vi "Process.vi"(8 "error in":errorcluster, 11 "Inst UI.Xeryon-Rotator":refnum<class "Inst UI.Xeryon-Rotator.lvclass">) -> (0 "error out":errorcluster, 3 "Inst UI.Xeryon-Rotator out":refnum<class "Inst UI.Xeryon-Rotator.lvclass">)   [LabVIEW 2019, in "Inst UI.Xeryon-Rotator.lvclass"]
doc: "---------------------------------------------------------------\nJKI State Machine Objects™\nhttp://jki.net/state-machine-objects/\nCopyright (C) 2005-2015, JKI <info@jki.net>\nALL RIGHTS RESERVEDJKI State Machine Objects (SMO) 1.0.0.5\nJKI - JKI\nCopyright (c) 2016, JKI"
uses:
  Inst UI.Xeryon-Rotator.lvclass
  C:/Program Files (x86)/National Instruments/LabVIEW 2019/vi.lib/JKI/JKI SMO/SMO/SMO.lvclass
  C:/Program Files (x86)/National Instruments/LabVIEW 2019/user.lib/LevyLab/Instrument Framework/Instrument UI/Instrument UI.lvclass
  C:/Program Files (x86)/National Instruments/LabVIEW 2019/vi.lib/JKI/JKI SMO/SMO.UI/SMO.UI.lvclass
  <userlib>/LevyLab/Instrument Framework/Instrument Types/Cryostat/Typedefs/setAngle--cluster.ctl
  Inst.Xeryon-Rotator/Typedefs/Inst.Xeryon-Rotator.ScanState--Enum.ctl
  Inst.Xeryon-Rotator/Typedefs/Inst.Xeryon-Rotator.getAll--Cluster.ctl
  Inst.Xeryon-Rotator/Inst.Xeryon-Rotator.lvclass
  C:/Program Files (x86)/National Instruments/LabVIEW 2019/user.lib/LevyLab/Instrument Framework/Instrument/Instrument.lvclass
  Inst UI.Xeryon-Rotator.UI--Cluster.ctl
  <userlib>/LevyLab/Configuration/Configuration.lvclass
  <userlib>/LevyLab/RemoteControl/RemoteControl/Typedefs/Message--Cluster.ctl
  <userlib>/LevyLab/Instrument Framework/Instrument UI/Instrument UI.lvclass/Instrument UI.ctl
  Inst.Xeryon-Rotator/Inst.Xeryon-Rotator.lvclass/Inst.Xeryon-Rotator.ctl
  <vilib>/JKI/JKI SMO/SMO/SMO.lvclass/SMO.ctl
  <userlib>/LevyLab/Configuration/Configuration.lvclass/Configuration.ctl
  <userlib>/LevyLab/Instrument Framework/Instrument/Typedefs/Client Type--Enum.ctl
  <userlib>/LevyLab/Instrument Framework/Instrument/Instrument.lvclass/Instrument.ctl
  e9f0865c-66ad-4c19-bb34-0e698946f1b4.vi
  fbc1e19e-d7b2-448f-8f6c-080fe6692cf7.vi
  2b403158-dc38-43e7-94d2-04ca50d476d7.vi
  2b5fa6da-c280-4914-92c0-3208c3c43a45.vi
  20157899-4549-4947-8324-d0895f4678d5.vi
  cd4b701c-744b-455d-abd0-f4a1a0a0dcf1.vi
  <vilib>/JKI/JKI SMO/SMO/Private/ReftoDVR--SMO.vi
  cd4b701c-744b-455d-abd0-f4a1a0a0dcf1.vi/5058294c-336d-4b2b-804e-8f9495cbe216.vi
  cd4b701c-744b-455d-abd0-f4a1a0a0dcf1.vi/49ec677a-2f26-4dd4-a9e7-83f22994531d.vi
  <vilib>/JDP Science/JSONtext/Variant to JSON Text.vi
  <vilib>/Utility/Data Type/Get Type Information.vi
  <vilib>/JDP Science/JSONtext/JSON text to Variant.vi
  <userlib>/LevyLab/Instrument Framework/Instrument/API/Instrument.sendMessageToProcess (string).vi
  <vilib>/JDP Science/JSONtext/LVClass Serializer/JSONtext LVClass Serializer.lvclass
  <userlib>/LevyLab/Instrument Framework/Instrument/Instrument.lvclass
  <userlib>/LevyLab/Instrument Framework/Instrument UI/Instrument UI.lvclass
  <userlib>/LevyLab/RemoteControl/RemoteControl/RemoteControl.lvclass
  C:/Program Files (x86)/National Instruments/LabVIEW 2019/user.lib/LevyLab/Instrument Framework/Instrument Types/Cryostat/Instrument.Cryostat.lvclass
  <userlib>/LevyLab/Instrument Framework/Instrument Types/Cryostat/Instrument.Cryostat.lvclass
  <vilib>/JKI/JKI SMO/SMO/SMO.lvclass
  <vilib>/JKI/JKI SMO/SMO.UI/SMO.UI.lvclass
panel:
  in  "Reset":bool
  out "STAT":string
  in  "Rotate Right":bool
  in  "Rotate Left":bool
  in  "Stop":bool
  out "Color Box":u32(colorbox)
  in  "Rate (°/min)":dbl=1000.0
  out "Waveform Chart":T1(graph)
  out "Position Reached":bool
  out "Right Limit":bool
  out "Left Limit":bool
  out "Index Found":bool
  out "Encoder Position (encoder units)":dbl format="%#_8f"
  out "Desired Position (encoder units)":dbl format="%#_8f"
  out "Encoder Position (°)":dbl
  out "Desired Position (°)":dbl
  out "Numeric":u32
  in  "Go To Position":bool
  in  "Desired Position (°)":dbl
  # "SMO UI Template"
  # "For instructions on how to use the JKI State Machine Objects, examples and video tutorials, visit:\nhttp://jki.net/state-machine-objects/\n\nJKI State Machine Objects™\nhttp://jki.net/state-machine-objects/\nCopyright (C) 2005-2015, JKI <info@jki.net>\nALL RIGHTS RESERVED"
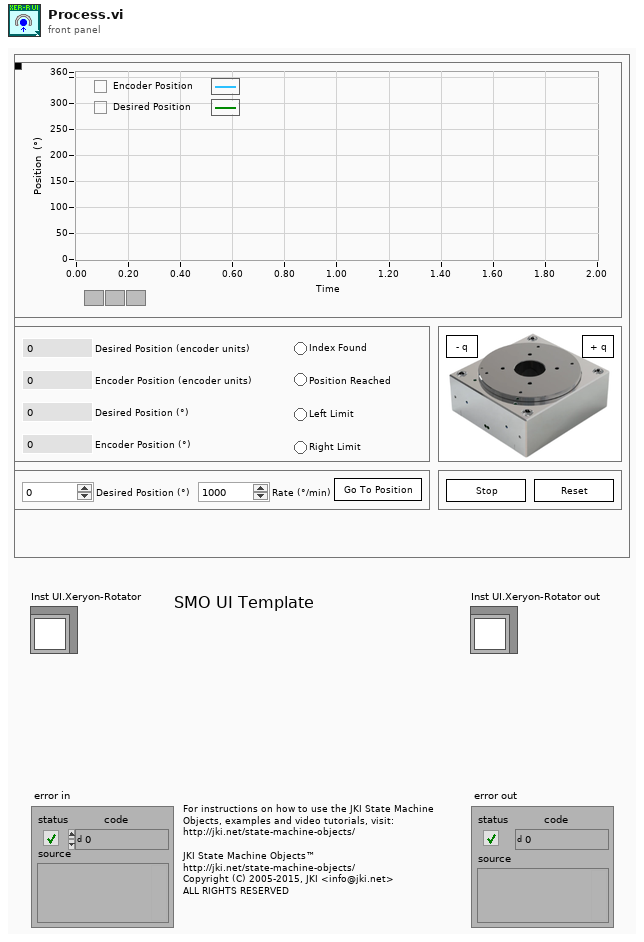
[diagram p1: front panel]
types:
  T1 = cluster{"DPOS In Current Units":dbl, "EPOS In Current Units":dbl}
  T2 = typedef "Instrument.Cryostat.lvclass/setAngle--cluster.ctl" = cluster{"angle":dbl, "rate":dbl, "channel":i32}
  T3 = typedef "Inst.Xeryon-Rotator.lvclass/Inst.Xeryon-Rotator.ScanState--Enum.ctl" = enum16{"Scan Left", "Stop", "Scan Right", "Reset"}
  T4 = enum32{"invalid app kind", "Development System", "Run Time System", "Student Edition", "Embedded LabVIEW", "Evaluation", "Custom"}
  T5 = typedef "Inst.Xeryon-Rotator.lvclass/Inst.Xeryon-Rotator.getAll--Cluster.ctl" = cluster{"Encoder position [selected units]":dbl, "Desired Position [selected units]":dbl, "Status":string, "SRNO":dbl, "SOFT":dbl, "STAT":dbl, "FREQ":dbl, "OFRQ":dbl, "CURR":dbl, "SYNC":dbl, "Encoder Position [enc. units]":dbl, "Desired Position [enc. units]":dbl, "TIME":dbl, "Index Found":bool, "Left Limit":bool, "Right Limit":bool, "Position Reached":bool}
  T6 = enum32{"Invalid", "Standard", "Closed", "Hidden", "Minimized", "Maximized"}
  T7 = typedef "Instrument.lvlib/Instrument.lvclass/Client Type--Enum.ctl" = enum16{"Remote", "Local"}
  T8 = typedef "Inst UI.Xeryon-Rotator.lvclass/Inst UI.Xeryon-Rotator.UI--Cluster.ctl" = cluster{"Desired Position":dbl, "Desired Rate":dbl}
  T9 = typedef "RemoteControl.lvlib/RemoteControl.lvclass/Message--Cluster.ctl" = cluster{"Command":string, "Data":variant, "ID":string, "error":errorcluster}
  T10 = cluster{"Core":cluster{"Current VI Reference":refnum<vi>, "Close Panel on Exit?":bool, "Last Error":cluster{"error":errorcluster, "previous state":string, "remaining states":string}, "Shutdown?":bool}, "Instrument UI":refnum<class "Inst UI.Xeryon-Rotator.lvclass">, "Instrument":refnum<class "Inst.Xeryon-Rotator.lvclass">, "Configuration":refnum<class "Configuration.lvclass">, "getAll":T5, "UI Cluster":T8, "Message":T9}
  T11 = cluster{"Current VI Reference":refnum<vi>, "Close Panel on Exit?":bool, "Last Error":cluster{"error":errorcluster, "previous state":string, "remaining states":string}, "Shutdown?":bool}
  T12 = cluster{"Encoder position [selected units]":dbl, "Desired Position [selected units]":dbl}
  T13 = typedef "SMO.lvclass/Protected Events.ctl" = cluster{"StopProcesses":refnum<user-event>, "AbortProcesses":refnum<user-event>, "Config Changed":refnum<user-event>, "Dependency":refnum<user-event>}
  T14 = typedef "Instrument.lvlib/Instrument.lvclass/PublicEvents--Cluster.ctl" = cluster{"MessageFromProcess":refnum<user-event>}
  T15 = typedef "Inst.Xeryon-Rotator.lvclass/PublicEvents--Cluster.ctl" = cluster{"MessageFromProcess":refnum<user-event>}
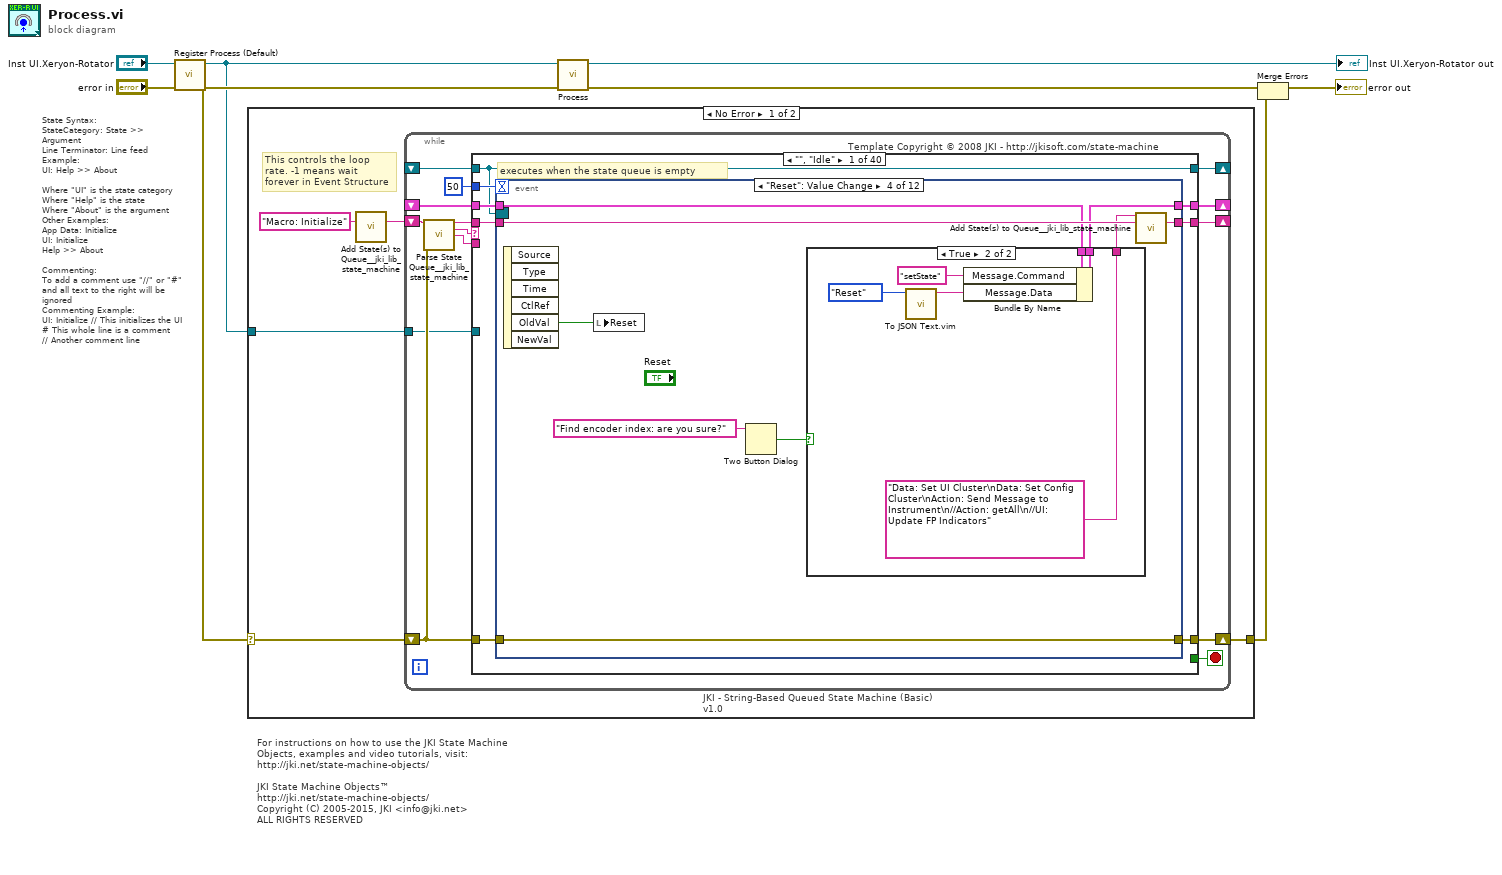
[diagram p0: block diagram]
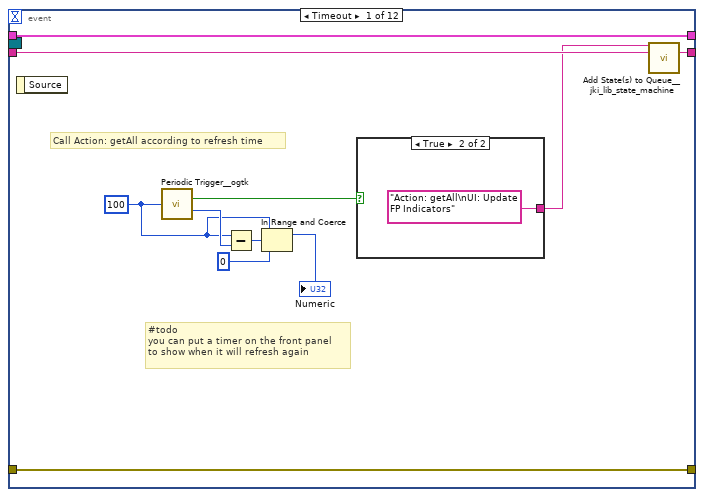
[diagram p2: hidden frame]
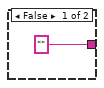
[diagram p3: hidden frame]
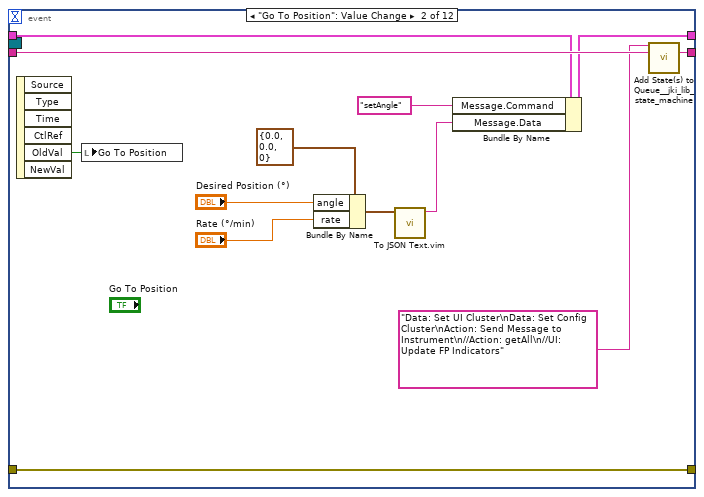
[diagram p4: hidden frame]
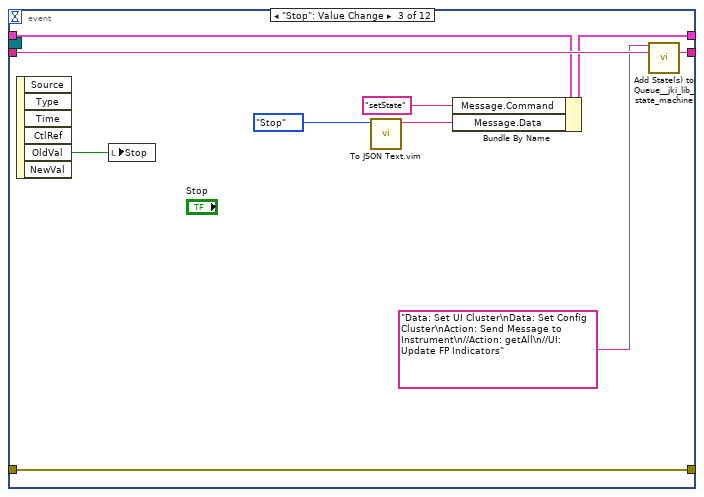
[diagram p5: hidden frame]
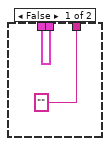
[diagram p6: hidden frame]
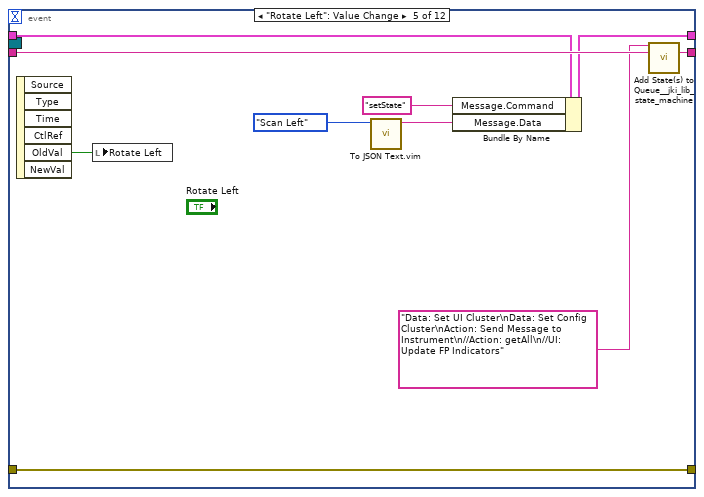
[diagram p7: hidden frame]
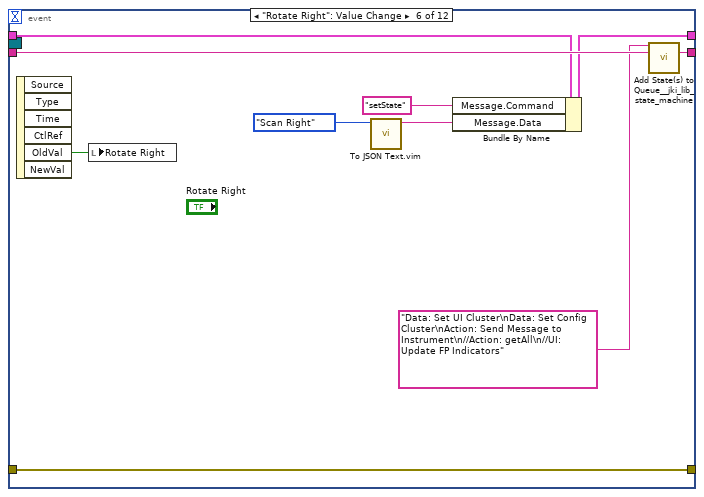
[diagram p8: hidden frame]
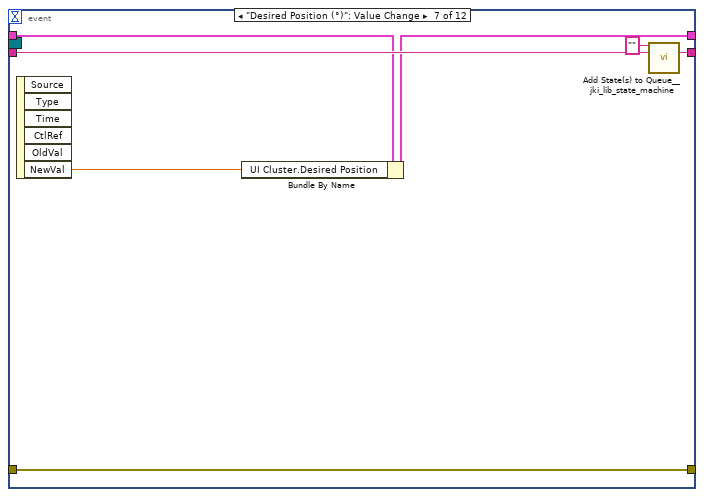
[diagram p9: hidden frame]
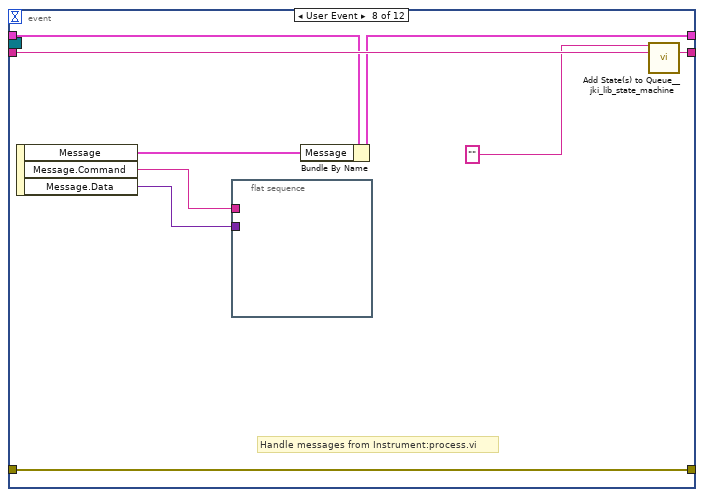
[diagram p10: hidden frame]
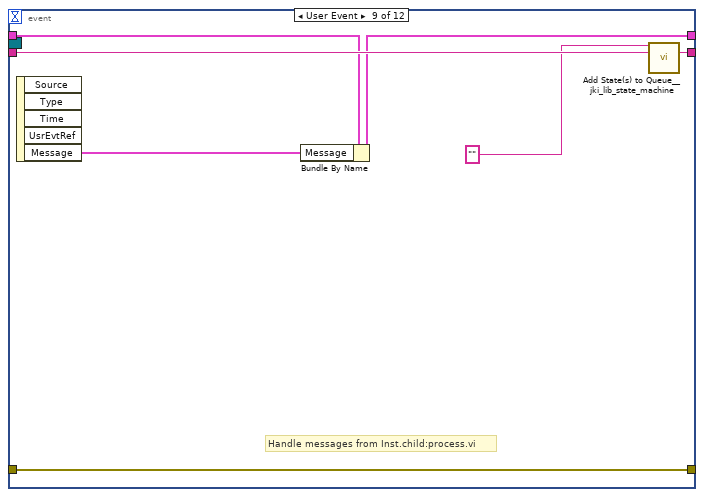
[diagram p11: hidden frame]
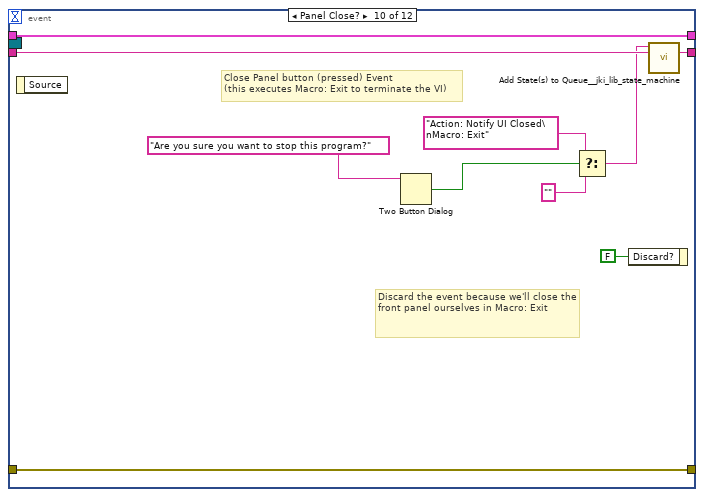
[diagram p12: hidden frame]
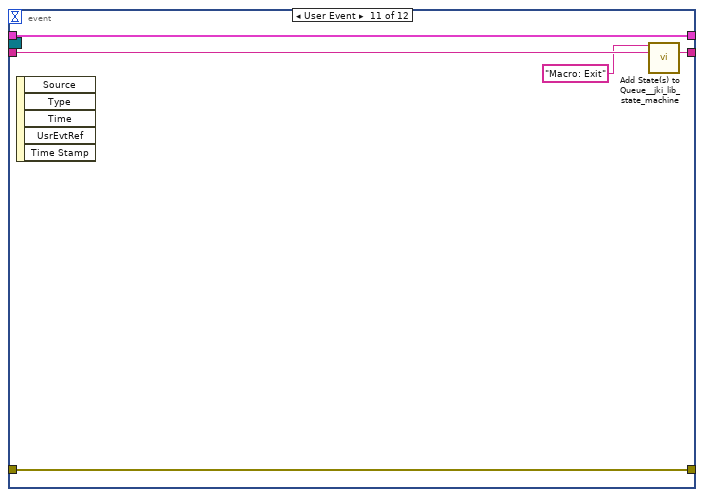
[diagram p13: hidden frame]
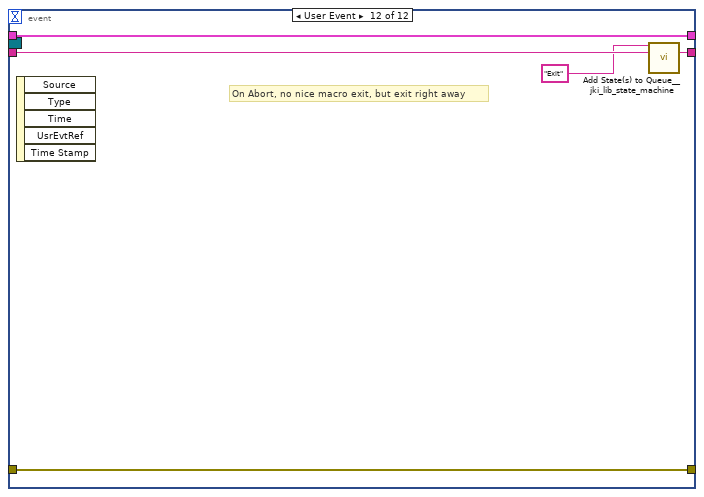
[diagram p14: hidden frame]
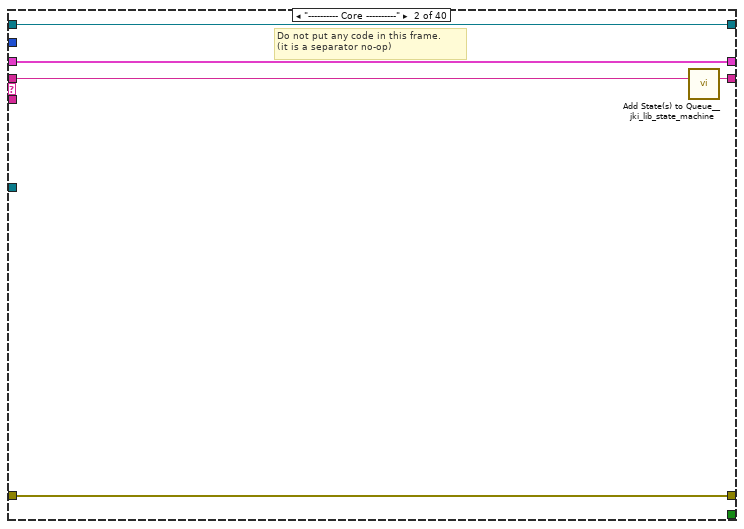
[diagram p15: hidden frame]
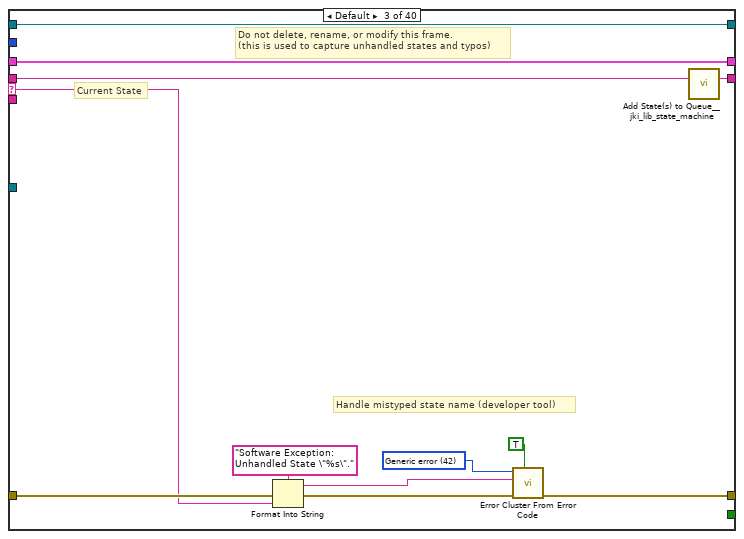
[diagram p16: hidden frame]
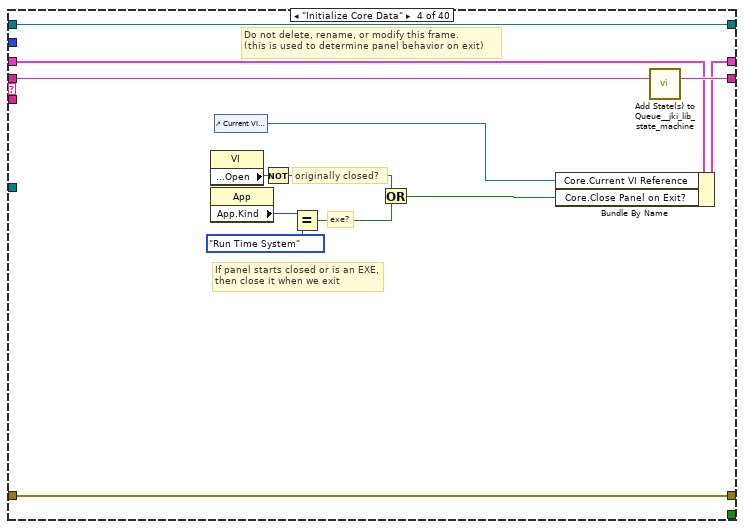
[diagram p17: hidden frame]
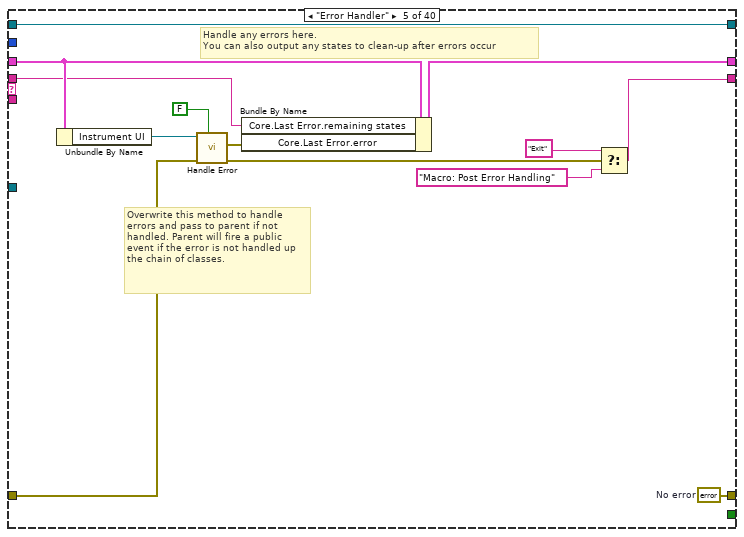
[diagram p18: hidden frame]
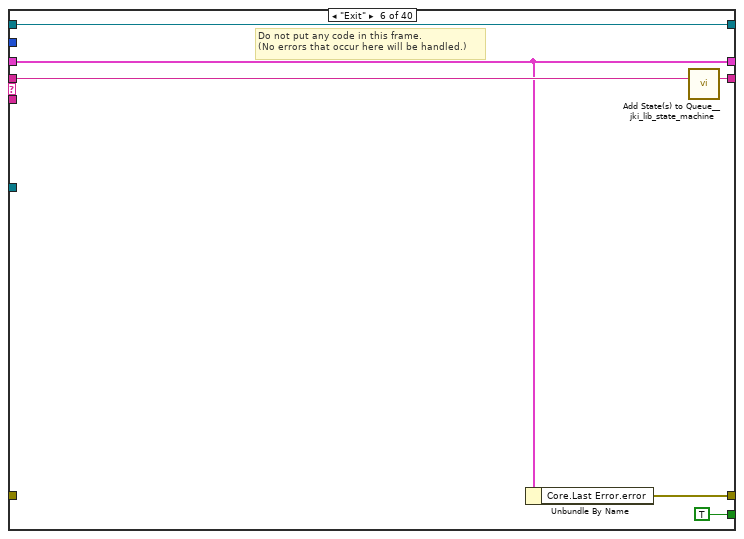
[diagram p19: hidden frame]
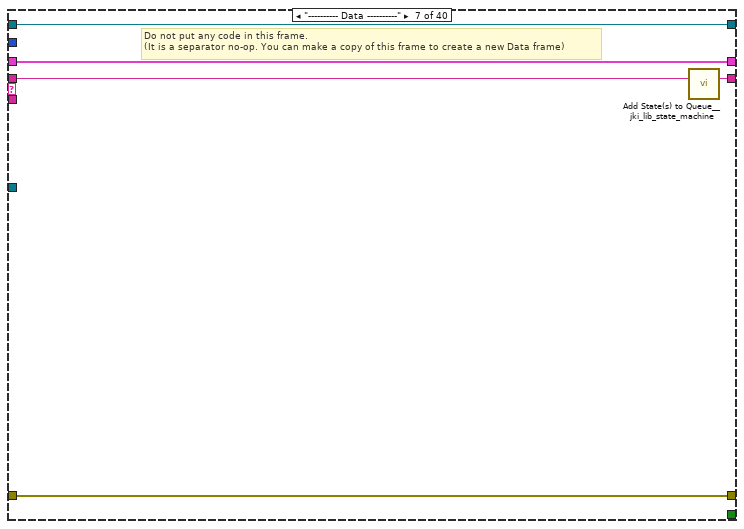
[diagram p20: hidden frame]
diagram:
  # "State Syntax:\nStateCategory: State >> Argument\nLine Terminator: Line feed\nExample:\nUI: Help >> About\n\nWhere \"UI\" is the state category\nWhere \"Help\" is the state\nWhere \"About\" is the argument\nOther Examples:\nApp Data: Initialize\nUI: Initialize\nHelp >> About\n\nCommenting:\nTo add a comment use \"//\" or \"#\" and all text to the right will be ignored\nCommenting Example:\nUI: Initialize // This initializes the UI\n# This whole line is a comment\n// Another comment line"
  # "For instructions on how to use the JKI State Machine Objects, examples and video tutorials, visit:\nhttp://jki.net/state-machine-objects/\n\nJKI State Machine Objects™\nhttp://jki.net/state-machine-objects/\nCopyright (C) 2005-2015, JKI <info@jki.net>\nALL RIGHTS RESERVED"
  n1 = call <vilib>:"Register Process (Default).vi"("error in (no error)"="error in", "SMO"="Inst UI.Xeryon-Rotator") -> ("error out"=w5:errorcluster, "SelfRef"=w4:refnum<class "Inst UI.Xeryon-Rotator.lvclass">)  [unwired: 8 in]
  n2 = case shown="No Error" w5 {
    selector: w5 -> [w10 w564]
    tunnel: w4 -> [w11 _]
    tunnel: [w9 w564] -> w1
    frame No Error {
      # "This controls the loop rate. -1 means wait forever in Event Structure"
      n3 = call <vilib>:"Add State(s) to Queue__jki_lib_state_machine.vi"("State(s) in (\"\")"="Macro: Initialize") -> ("States Out"=w13:string)  [unwired: 14 in]
      n4 = while "JKI - String-Based Queued State Machine (Basic) v1.0" {
        shift-right: [w20] -> _
        shift-left: _ -> [w19]
        shift-right: [w23] -> w9
        shift-left: w10 -> [w17]
        shift-right: [w22] -> _
        shift-left: w13 -> [w24]
        tunnel: w11 -> [w16]
        shift-right: [w15] -> _
        shift-left: _ -> [w14]
        stop <- w21 stop-if-true
        # "Template Copyright © 2008 JKI - http://jkisoft.com/state-machine"
        n5 = call <vilib>:"Parse State Queue__jki_lib_state_machine.vi"("State Queue"=w24, "Error In (no error)"=w17) -> ("Remaining States"=w26:string, "Current State"=w27:string, "Arguments"=w25:string)  [unwired: 11 in]
        n6 = case shown="\"\", \"Idle\"" w27 {
          selector: w27 -> [_ _ w158 _ _ _ _ _ _ _ _ _ _ _ _ _ _ _ _ _ _ _ _ _ _ _ _ _ _ _ _ _ _ _ _ _ _ _ _ _]
          tunnel: w26 -> [w35 w156 w162 w181 w185 w200 w205 w222 w230 w238 w245 w250 w257 w264 w272 w298 w314 w346 w355 w367 w377 w383 w398 w403 w414 w421 w426 w442 w448 w453 w468 w476 w488 w495 w502 w516 w529 w539 w551 w563]
          tunnel: w25 -> [_ _ _ _ _ _ _ _ _ _ _ _ _ _ _ w292 w308 _ _ _ _ _ _ _ _ _ _ _ _ _ _ _ _ _ _ _ _ _ _ _]
          tunnel: w19 -> [w33 w153 w160 w172 w188 w196 w202 _ w226 w234 w239 w247 w255 w260 w268 w296 w310 w343 w351 w357 w374 w380 w385 w400 w411 w416 w423 w440 w446 w450 w461 w473 w479 w490 w496 w509 w523 w531 w546 w558]
          tunnel: [w32 w154 w164 w178 w190 w195 w203 w210 w228 w236 w241 w248 w252 w262 w269 w293 w311 w344 w353 w365 w375 w381 w396 w401 w405 w417 w424 w437 w443 w451 w454 w471 w480 w492 w497 w503 w526 w536 w542 w554] -> w23
          tunnel: w17 -> [w31 w154 w163 w178 w184 _ w203 w207 w228 w236 w242 w248 w253 w262 w269 w294 w312 w344 w353 w365 w375 w381 w396 w401 w406 w418 w424 w427 w444 w451 w463 w469 w481 w492 w498 w510 w518 w532 w543 w555]
          tunnel: [w34 w155 w161 w180 w182 w199 w204 w221 w229 w237 w244 w249 w256 w263 w271 w297 w313 w345 w354 w366 w376 w382 w397 w402 w413 w420 w425 w441 w447 w452 w467 w475 w487 w494 w501 w515 w528 w538 w550 w562] -> w22
          tunnel: [_ _ _ _ _ TRUE _ _ _ _ _ _ _ _ _ _ _ _ _ _ _ _ _ _ _ _ _ _ _ _ _ _ _ _ _ _ _ _ _ _] -> w21
          tunnel: [w30 w153 w160 w179 w187 w196 w202 w220 w225 w233 w239 w247 w255 w260 w268 w296 w310 w343 w351 w358 w374 w380 w385 w400 w411 w416 w423 w440 w446 w450 w465 w473 w477 w489 w496 w511 w524 w533 w547 w559] -> w20
          tunnel: 50 ("Timeout") -> [w29 _ _ _ _ _ _ _ _ _ _ _ _ _ _ _ _ _ _ _ _ _ _ _ _ _ _ _ _ _ _ _ _ _ _ _ _ _ _ _]
          tunnel: w16 -> [_ _ _ _ _ _ _ w208 _ _ _ _ _ _ _ _ _ _ _ _ _ _ _ _ _ _ _ _ _ _ _ _ _ _ _ _ _ _ _ _]
          tunnel: [w28 w152 w157 w169 w194 w197 w201 w219 w227 w235 w240 w246 w254 w261 w270 w295 w307 w342 w352 w364 w373 w379 w390 w399 w412 w419 w422 w439 w445 w449 w466 w474 w486 w493 w500 w514 w527 w537 w549 w561] -> w15
          tunnel: w14 -> [w28 w152 w157 w169 w194 w197 w201 w219 w227 w235 w240 w246 w254 w261 w270 w295 w307 w342 w352 w364 w373 w379 w390 w399 w412 w419 w422 _ w445 w449 w466 w474 w486 w493 w500 w514 w527 w537 w549 w561]
          frame "", "Idle" {
            # "executes when the state queue is empty"
            n7 = event shown="[3] \"Reset\": Value Change" {
              selector: w28 -> [_ _ _ _ _ _ _ _ _ _ _ _]
              dyn-events: _ -> [_ _ _ _ _ _ _ _ _ _ _ _]
              timeout: w29 -> [_ _ _ _ _ _ _ _ _ _ _ _]
              tunnel: w35 -> [w46 w61 w71 w80 w98 w108 w115 w124 w131 w141 w146 w151]
              tunnel: [w45 w60 w70 w79 w97 w107 w114 w123 w130 w140 w145 w150] -> w34
              tunnel: w33 -> [w43 w55 w65 w74 w92 w102 w111 w121 w128 w138 w143 w148]
              tunnel: [w44 w59 w69 w78 w96 w106 w113 w122 w129 w137 w144 w149] -> w32
              tunnel: w31 -> [w44 w59 w69 w78 w96 w106 w113 w122 w129 w137 w144 w149]
              tunnel: [w43 w56 w66 w75 w93 w103 w110 w120 w127 w138 w143 w148] -> w30
              event Timeout {
                w37 = u32 100 ("time (ms)")
                # "#todo\nyou can put a timer on the front panel\nto show when it will refresh again"
                # "Call Action: getAll according to refresh time"
                n8 = event-data() -> ()  [unwired: 1 in, 1 out]
                n9 = call <userlib>:"Periodic Trigger__ogtk.vi"("time (ms)"=w37) -> ("Triggered"=w41:bool, "timer value"=w40:u32)  [unwired: 12 in, 1 out]
                n10 = Subtract(x=w37, y=w40) -> (x-y=w39:u32)
                n11 = In Range and Coerce(upper limit=w37, x=w39, lower limit=u32 0) -> (coerced(x)=→"Numeric":u32)  [unwired: 1 out]
                n12 = case shown="True" w41 {
                  tunnel: ["" ("State(s) in Front (\"\")") "Action: getAll\nUI: Update FP Indicators" ("State(s) in Front (\"\")")] -> w42
                  frame False {
                  }
                  frame True {
                  }
                }
                n13 = call <vilib>:"Add State(s) to Queue__jki_lib_state_machine.vi"("State(s) in Front (\"\")"=w42, "State(s) in (\"\")"=w46) -> ("States Out"=w45:string)  [unwired: 13 in]
              }
              event "Go To Position": Value Change {
                n14 = event-data() -> ("OldVal"=w58:bool)  [unwired: 1 in, 5 out]
                n15 = local write "Go To Position"(w58) -> ()
                n16 = Bundle By Name(cluster=T2 {"angle"=0.0, "rate"=0.0, "channel"=0} ("setAngle"), "angle"="Desired Position (°)", "rate"="Rate (°/min)") -> (w50:T2)
                n17 = call "To JSON Text.vim"("Anything"=w50) -> ("<JSON>"=w49:string)  [unwired: 9 in, 1 out]
                n18 = Bundle By Name(cluster=w55, "Message.Command"="setAngle", "Message.Data"=w49) -> (w56:T10)
                n19 = call <vilib>:"Add State(s) to Queue__jki_lib_state_machine.vi"("State(s) in Front (\"\")"="Data: Set UI Cluster\nData: Set Config Cluster\nAction: Send Message to Instrument\n//Action: getAll\n//UI: Update FP Indicators" ("State(s) in Front (\"\")"), "State(s) in (\"\")"=w61) -> ("States Out"=w60:string)  [unwired: 13 in]
              }
              event "Stop": Value Change {
                n20 = event-data() -> ("OldVal"=w68:bool)  [unwired: 1 in, 5 out]
                n21 = local write "Stop"(w68) -> ()
                n22 = call "To JSON Text.vim"("Anything"=Inst.Xeryon-Rotator.ScanState--Enum."Stop" ("Scan State")) -> ("<JSON>"=w63:string)  [unwired: 9 in, 1 out]
                n23 = Bundle By Name(cluster=w65, "Message.Command"="setState", "Message.Data"=w63) -> (w66:T10)
                n24 = call <vilib>:"Add State(s) to Queue__jki_lib_state_machine.vi"("State(s) in Front (\"\")"="Data: Set UI Cluster\nData: Set Config Cluster\nAction: Send Message to Instrument\n//Action: getAll\n//UI: Update FP Indicators" ("State(s) in Front (\"\")"), "State(s) in (\"\")"=w71) -> ("States Out"=w70:string)  [unwired: 13 in]
              }
              event "Reset": Value Change {
                n25 = event-data() -> ("OldVal"=w77:bool)  [unwired: 1 in, 5 out]
                n26 = local write "Reset"(w77) -> ()
                n27 = Two Button Dialog(message="Find encoder index: are you sure?") -> (T button?=w72:bool)  [unwired: 2 in]
                n28 = case shown="True" w72 {
                  tunnel: ["" ("State(s) in Front (\"\")") "Data: Set UI Cluster\nData: Set Config Cluster\nAction: Send Message to Instrument\n//Action: getAll\n//UI: Update FP Indicators" ("State(s) in Front (\"\")")] -> w76
                  tunnel: [w82 w87] -> w75
                  tunnel: w74 -> [w82 w86]
                  frame False {
                  }
                  frame True {
                    n29 = call "To JSON Text.vim"("Anything"=Inst.Xeryon-Rotator.ScanState--Enum."Reset" ("Scan State")) -> ("<JSON>"=w84:string)  [unwired: 9 in, 1 out]
                    n30 = Bundle By Name(cluster=w86, "Message.Command"="setState", "Message.Data"=w84) -> (w87:T10)
                  }
                }
                n31 = call <vilib>:"Add State(s) to Queue__jki_lib_state_machine.vi"("State(s) in Front (\"\")"=w76, "State(s) in (\"\")"=w80) -> ("States Out"=w79:string)  [unwired: 13 in]
              }
              event "Rotate Left": Value Change {
                n32 = event-data() -> ("OldVal"=w95:bool)  [unwired: 1 in, 5 out]
                n33 = local write "Rotate Left"(w95) -> ()
                n34 = call "To JSON Text.vim"("Anything"=Inst.Xeryon-Rotator.ScanState--Enum."Scan Left" ("Scan State")) -> ("<JSON>"=w90:string)  [unwired: 9 in, 1 out]
                n35 = Bundle By Name(cluster=w92, "Message.Command"="setState", "Message.Data"=w90) -> (w93:T10)
                n36 = call <vilib>:"Add State(s) to Queue__jki_lib_state_machine.vi"("State(s) in Front (\"\")"="Data: Set UI Cluster\nData: Set Config Cluster\nAction: Send Message to Instrument\n//Action: getAll\n//UI: Update FP Indicators" ("State(s) in Front (\"\")"), "State(s) in (\"\")"=w98) -> ("States Out"=w97:string)  [unwired: 13 in]
              }
              event "Rotate Right": Value Change {
                n37 = event-data() -> ("OldVal"=w105:bool)  [unwired: 1 in, 5 out]
                n38 = local write "Rotate Right"(w105) -> ()
                n39 = call "To JSON Text.vim"("Anything"=Inst.Xeryon-Rotator.ScanState--Enum."Scan Right" ("Scan State")) -> ("<JSON>"=w100:string)  [unwired: 9 in, 1 out]
                n40 = Bundle By Name(cluster=w102, "Message.Command"="setState", "Message.Data"=w100) -> (w103:T10)
                n41 = call <vilib>:"Add State(s) to Queue__jki_lib_state_machine.vi"("State(s) in Front (\"\")"="Data: Set UI Cluster\nData: Set Config Cluster\nAction: Send Message to Instrument\n//Action: getAll\n//UI: Update FP Indicators" ("State(s) in Front (\"\")"), "State(s) in (\"\")"=w108) -> ("States Out"=w107:string)  [unwired: 13 in]
              }
              event "Desired Position (°)": Value Change {
                n42 = event-data() -> ("NewVal"=w112:dbl)  [unwired: 1 in, 5 out]
                n43 = Bundle By Name(cluster=w111, "UI Cluster.Desired Position"=w112) -> (w110:T10)
                n44 = call <vilib>:"Add State(s) to Queue__jki_lib_state_machine.vi"("State(s) in Front (\"\")"="" ("State(s) in Front (\"\")"), "State(s) in (\"\")"=w115) -> ("States Out"=w114:string)  [unwired: 13 in]
              }
              event User Event {
                # "Handle messages from Instrument:process.vi"
                n45 = event-data() -> ("Message"=w118:T9, "Message.Command"=w117:string, "Message.Data"=w116:variant)  [unwired: 1 in]
                n46 = flat-sequence {
                  tunnel: w117 -> [_]
                  tunnel: w116 -> [_]
                  frame #0 {
                  }
                }
                n47 = Bundle By Name(cluster=w121, "Message"=w118) -> (w120:T10)
                n48 = call <vilib>:"Add State(s) to Queue__jki_lib_state_machine.vi"("State(s) in Front (\"\")"="" ("State(s) in Front (\"\")"), "State(s) in (\"\")"=w124) -> ("States Out"=w123:string)  [unwired: 13 in]
              }
              event User Event {
                # "Handle messages from Inst.child:process.vi"
                n49 = event-data() -> ("Message"=w125:T9)  [unwired: 1 in, 4 out]
                n50 = Bundle By Name(cluster=w128, "Message"=w125) -> (w127:T10)
                n51 = call <vilib>:"Add State(s) to Queue__jki_lib_state_machine.vi"("State(s) in Front (\"\")"="" ("State(s) in Front (\"\")"), "State(s) in (\"\")"=w131) -> ("States Out"=w130:string)  [unwired: 13 in]
              }
              event Panel Close? {
                # "Discard the event because we'll close the front panel ourselves in Macro: Exit"
                # "Close Panel button (pressed) Event\n(this executes Macro: Exit to terminate the VI)"
                n52 = event-data() -> ()  [unwired: 1 in, 1 out]
                n53 = Two Button Dialog(message="Are you sure you want to stop this program?") -> (T button?=w136:bool)  [unwired: 2 in]
                n54 = Select(t="Action: Notify UI Closed\nMacro: Exit", s=w136, f="") -> (s? t:f=w132:string)
                n55 = event-data("Discard?"=FALSE) -> ()  [unwired: 1 in, 1 out]
                n56 = call <vilib>:"Add State(s) to Queue__jki_lib_state_machine.vi"("State(s) in Front (\"\")"=w132, "State(s) in (\"\")"=w141) -> ("States Out"=w140:string)  [unwired: 13 in]
              }
              event User Event {
                n57 = event-data() -> ()  [unwired: 1 in, 5 out]
                n58 = call <vilib>:"Add State(s) to Queue__jki_lib_state_machine.vi"("State(s) in Front (\"\")"="Macro: Exit", "State(s) in (\"\")"=w146) -> ("States Out"=w145:string)  [unwired: 13 in]
              }
              event User Event {
                # "On Abort, no nice macro exit, but exit right away"
                n59 = event-data() -> ()  [unwired: 1 in, 5 out]
                n60 = call <vilib>:"Add State(s) to Queue__jki_lib_state_machine.vi"("State(s) in Front (\"\")"="Exit", "State(s) in (\"\")"=w151) -> ("States Out"=w150:string)  [unwired: 13 in]
              }
            }
          }
          frame "---------- Core ----------" {
            # "Do not put any code in this frame.\n(it is a separator no-op)"
            n61 = call <vilib>:"Add State(s) to Queue__jki_lib_state_machine.vi"("State(s) in (\"\")"=w156) -> ("States Out"=w155:string)  [unwired: 14 in]
          }
          frame Default {
            w167 = 42 items=["No error", "Argument error", "Memory is full", "Out of zone", "End of file", "File already open", "Generic file I/O error", "File not found", "File permission error", "Disk is full", "Duplicate path", "Too many files open", "System feature not enabled", "Resource file not found", "Cannot add resource", "Resource not found", "Image not found", "Image memory error", "Pen does not exist", "Config type invalid", "Config token not found", "Config parse error", "Config memory error", "Bad external code format", "Bad external code offset", "External code not present", "Null window", "Destroy window error", "Null menu", "Print aborted", "Bad print record", "Print driver error", "Windows error during printing", "Memory error during printing", "Print dialog error", "Generic print error", "Invalid device refnum", "Device not found", "Device parameter error", "Device unit error", "Cannot open device", "Device call aborted", "Generic error", "Cancelled by user", "Object ID too low", "Object ID too high", "Object not in heap", "Unknown heap", "Unknown object (invalid DefProc)", "Unknown object (DefProc not in table)", "Message out of range", "Invalid (null) method", "Unknown message", "Manager call not supported", "Bad address", "Network operation in progress", "Network operation timed out", "Connection is busy", "Network attribute not supported", "Network error", "Address in use", "System out of memory", "Connection aborted", "Connection refused", "Not connected", "Already connected", "Connection closed", "Initialization error (interapplication manager)", "Bad occurrence", "Wait on unbound occurrence handler", "Occurrence queue overflow", "Datalog type conflict", "Unused", "Unrecognized type (interapplication manager)", "Memory corrupt", "Failed to make temporary DLL", "Old CIN version", "Drag socket not found", "Failed to load drop-object", "Failed to register OLE object", "Failed to release OLE object", "Format specifier type mismatch", "Unknown format specifier", "Too few format specifiers", "Too many format specifiers", "Scan failed", "Newer CIN version", "Error converting to variant", "Runtime menu error", "Password tampered", "Variant attribute not found", "Incompatible variant data type", "Event data is not available", "Event Store is not present", "Occurrence is not found", "Event Queue is not created", "Event info is not available", "Refnum passed is NULL", "Error retrieving Class GUID", "Error retrieving CoClass GUID", "Error retrieving TypeLib GUID.", "Bad built application magic bytes.", "Specific driver is different from the specific driver associated with the Logical Name.", "There is no session opened to the class driver.", "Max Error", "MAX - Error with config objects", "MAX - Error loading configuration", "MAX - Group not supported"]
            # "Current State"
            # "Do not delete, rename, or modify this frame.\n(this is used to capture unhandled states and typos)"
            # "Handle mistyped state name (developer tool)"
            n62 = Format Into String(format string="Software Exception: Unhandled State \"%s\"." ("message"), error in=w163, w158) -> (resulting string=w166:string, error out=w165:errorcluster)  [unwired: 1 in]
            n63 = call <vilib>:"Error Cluster From Error Code.vi"("show call chain? (False)"=TRUE, "error in (no error)"=w165, "error message (\"\")"=w166, "error code (0)"=w167) -> ("error out"=w164:errorcluster)  [unwired: 5 in]
            n64 = call <vilib>:"Add State(s) to Queue__jki_lib_state_machine.vi"("State(s) in (\"\")"=w162) -> ("States Out"=w161:string)  [unwired: 14 in]
          }
          frame "Initialize Core Data" {
            # "Do not delete, rename, or modify this frame.\n(this is used to determine panel behavior on exit)"
            # "originally closed?"
            # "exe?"
            # "If panel starts closed or is an EXE, then close it when we exit"
            n65 = property class="VI"() -> ("Front Panel.Open"=w177:bool)  [unwired: 2 in, 2 out]
            n66 = property class="App"() -> ("App.Kind"=w176:T4)  [unwired: 2 in, 2 out]
            n67 = control-ref of="Current VI Reference"() -> (w170:refnum<vi>)
            n68 = Not(x=w177) -> (.not. x?=w174:bool)
            n69 = Equal?(x=w176, y=T4."Run Time System" ("Application:Kind")) -> (x = y?=w173:bool)
            n70 = Or(x=w174, y=w173) -> (x .or. y?=w171:bool)
            n71 = Bundle By Name(cluster=w172, "Core.Current VI Reference"=w170, "Core.Close Panel on Exit?"=w171) -> (w179:T10)
            n72 = call <vilib>:"Add State(s) to Queue__jki_lib_state_machine.vi"("State(s) in (\"\")"=w181) -> ("States Out"=w180:string)  [unwired: 14 in]
          }
          frame "Error Handler" {
            w190 = errorcluster {"status"=FALSE, "code"=0, "source"=""}  # No error
            # "Overwrite this method to handle errors and pass to parent if not handled. Parent will fire a public event if the error is not handled up the chain of classes."
            # "Handle any errors here.\nYou can also output any states to clean-up after errors occur"
            n73 = Unbundle By Name(w188) -> ("Instrument UI"=w193:refnum<class "Inst UI.Xeryon-Rotator.lvclass">)
            n74 = call-dynamic "Handle Error.vi"("Stop on Unhandled Error (T)"=FALSE, "error in"=w184, "SMO"=w193) -> ("handling error"=w191:errorcluster, "Unhandled error"=w189:errorcluster)  [unwired: 6 in, 1 out]
            n75 = Bundle By Name(cluster=w188, "Core.Last Error.remaining states"=w185, "Core.Last Error.error"=w189) -> (w187:T10)
            n76 = Select(t="Exit", s=w191, f="Macro: Post Error Handling") -> (s? t:f=w182:string)
          }
          frame "Exit" {
            # "Do not put any code in this frame.\n(No errors that occur here will be handled.)"
            n77 = Unbundle By Name(w196) -> ("Core.Last Error.error"=w195:errorcluster)
            n78 = call <vilib>:"Add State(s) to Queue__jki_lib_state_machine.vi"("State(s) in (\"\")"=w200) -> ("States Out"=w199:string)  [unwired: 14 in]
          }
          frame "---------- Data ----------" {
            # "Do not put any code in this frame.\n(It is a separator no-op. You can make a copy of this frame to create a new Data frame)"
            n79 = call <vilib>:"Add State(s) to Queue__jki_lib_state_machine.vi"("State(s) in (\"\")"=w205) -> ("States Out"=w204:string)  [unwired: 14 in]
          }
          frame "Data: Initialize" {
            w206 = T9 {"Command"="", "Data"=variant, "ID"="", "error"={"status"=FALSE, "code"=0, "source"=""}}  # Message
            w209 = refnum<class "Configuration.lvclass"> refnum  # Configuration
            w213 = T8 {"Desired Position"=0.0, "Desired Rate"=0.0}  # UI Cluster
            w215 = refnum<class "Inst.Xeryon-Rotator.lvclass"> refnum  # Instrument
            w217 = T5 {"Encoder position [selected units]"=0.0, "Desired Position [selected units]"=0.0, "Status"="", "SRNO"=0.0, "SOFT"=0.0, "STAT"=0.0, "FREQ"=0.0, "OFRQ"=0.0, "CURR"=0.0, "SYNC"=0.0, "Encoder Position [enc. units]"=0.0, "Desired Position [enc. units]"=0.0, "TIME"=0.0, "Index Found"=FALSE, "Left Limit"=FALSE, "Right Limit"=FALSE, "Position Reached"=FALSE}  # getAll
            w218 = T11 {"Current VI Reference"=refnum, "Close Panel on Exit?"=FALSE, "Last Error"={"error"={"status"=FALSE, "code"=0, "source"=""}, "previous state"="", "remaining states"=""}, "Shutdown?"=FALSE}  # Core
            # "Cluster of UI\ninformation you\nwant to save/load"
            # "Child Instrument"
            # "typedef from Child Instrument"
            # "do not delete - used by framework"
            # "Data names and types of shift register data are defined by this bundle."
            # "Initialize the shift-register data, here.\n(data names are defined by what you wire into the bundle function)"
            n80 = call <userlib>:"Read Instrument.vi"("error in (no error)"=w207, "Instrument UI in"=w208) -> ("error out"=w212:errorcluster, "Instrument"=w214:refnum<class "Instrument.lvclass">, "Instrument UI"=w216:refnum<class "Inst UI.Xeryon-Rotator.lvclass">)  [unwired: 7 in]
            n81 = To More Specific Class(target class=w215, reference=w214, error in=w212) -> (specific class reference=w211:refnum<class "Inst.Xeryon-Rotator.lvclass">, error out=w210:errorcluster)
            n82 = Bundle("Core"=w218, "Instrument UI"=w216, "Instrument"=w211, "Configuration"=w209, "getAll"=w217, "UI Cluster"=w213, "Message"=w206) -> (w220:T10)  [unwired: 1 in]
            n83 = call <vilib>:"Add State(s) to Queue__jki_lib_state_machine.vi"("State(s) in (\"\")"=w222) -> ("States Out"=w221:string)  [unwired: 14 in]
          }
          frame "Data: Set UI Cluster" {
            # "Do not put any code in this frame.\n(It is a separator no-op. You can make a copy of this frame to create a new Data frame)"
            n84 = local read "Desired Position (°)"() -> (w224:dbl)
            n85 = local read "Rate (°/min)"() -> (w223:dbl)
            n86 = Bundle By Name(cluster=w226, "UI Cluster.Desired Position"=w224, "UI Cluster.Desired Rate"=w223) -> (w225:T10)
            n87 = call <vilib>:"Add State(s) to Queue__jki_lib_state_machine.vi"("State(s) in (\"\")"=w230) -> ("States Out"=w229:string)  [unwired: 14 in]
          }
          frame "Data: Set Config Cluster" {
            # "Do not put any code in this frame.\n(It is a separator no-op. You can make a copy of this frame to create a new Data frame)"
            n88 = Unbundle By Name(w234) -> ("UI Cluster.Desired Position"=w232:dbl)
            n89 = Square(x=w232) -> (x^2=w231:dbl)
            n90 = Bundle By Name(cluster=w234, "getAll.Encoder position [selected units]"=w232, "getAll.Desired Position [selected units]"=w231) -> (w233:T10)
            n91 = call <vilib>:"Add State(s) to Queue__jki_lib_state_machine.vi"("State(s) in (\"\")"=w238) -> ("States Out"=w237:string)  [unwired: 14 in]
          }
          frame "Data: Cleanup" {
            # "Cleanup any data and references, here.\n(this is called automatically, by the Macro: Exit)"
            n92 = Unbundle By Name(w239) -> ("Core.Current VI Reference"=w243:refnum<vi>)
            n93 = Close Reference(reference=w243, error in (no error)=w242) -> (error out=w241:errorcluster)
            n94 = call <vilib>:"Add State(s) to Queue__jki_lib_state_machine.vi"("State(s) in (\"\")"=w245) -> ("States Out"=w244:string)  [unwired: 14 in]
          }
          frame "---------- UI ----------" {
            # "Do not put any code in this frame.\n(It is a separator no-op. You can make a copy of this frame to create a new UI frame)"
            n95 = call <vilib>:"Add State(s) to Queue__jki_lib_state_machine.vi"("State(s) in (\"\")"=w250) -> ("States Out"=w249:string)  [unwired: 14 in]
          }
          frame "UI: Initialize" {
            # "size window to decoration box on front panel"
            # "Initialize the User Interface, here.\n(this is called automatically, by the Macro: Init)"
            n96 = call <userlib>:"Fit VI window to Largest Dec__ogtk.vi"("error in (no error)"=w253, "border spacing (2 px)"=0) -> ("error out"=w252:errorcluster)  [unwired: 4 in, 1 out]
            n97 = call <vilib>:"Add State(s) to Queue__jki_lib_state_machine.vi"("State(s) in (\"\")"=w257) -> ("States Out"=w256:string)  [unwired: 14 in]
          }
          frame "UI: Update FP Controls" {
            # "Do not put any code in this frame.\n(It is a separator no-op. You can make a copy of this frame to create a new UI frame)"
            n98 = Unbundle By Name(w260) -> ("UI Cluster.Desired Position"=w259:dbl, "UI Cluster.Desired Rate"=w258:dbl)
            n99 = local write "Desired Position (°)"(w259) -> ()
            n100 = local write "Rate (°/min)"(w258) -> ()
            n101 = call <vilib>:"Add State(s) to Queue__jki_lib_state_machine.vi"("State(s) in (\"\")"=w264) -> ("States Out"=w263:string)  [unwired: 14 in]
          }
          frame "UI: Update FP Indicators" {
            n102 = Unbundle By Name(w268) -> ("getAll"=w267:T5)
            n103 = Not Equal?(x=T5 {"Encoder position [selected units]"=0.0, "Desired Position [selected units]"=0.0, "Status"="", "SRNO"=0.0, "SOFT"=0.0, "STAT"=0.0, "FREQ"=0.0, "OFRQ"=0.0, "CURR"=0.0, "SYNC"=0.0, "Encoder Position [enc. units]"=0.0, "Desired Position [enc. units]"=0.0, "TIME"=0.0, "Index Found"=FALSE, "Left Limit"=FALSE, "Right Limit"=FALSE, "Position Reached"=FALSE} ("getAll"), y=w267) -> (x != y?=w265:bool)
            n104 = case shown="True" w265 {
              tunnel: w267 -> [_ w273]
              frame False {
              }
              frame True {
                # "do this way to have nicer UI or only display what you want"
                n105 = Unbundle By Name(w273) -> ("STAT"=w276:dbl, "Encoder Position [enc. units]"=→"Encoder Position (encoder units)":dbl, "Desired Position [enc. units]"=→"Desired Position (encoder units)":dbl, "TIME"=w281:dbl, "Desired Position [selected units]"=w278:dbl, "Encoder position [selected units]"=w279:dbl, "Index Found"=→"Index Found":bool, "Left Limit"=→"Left Limit":bool, "Right Limit"=→"Right Limit":bool, "Position Reached"=→"Position Reached":bool)  [unwired: 7 out]
                "Desired Position (°)" <- w278
                "Encoder Position (°)" <- w279
                n106 = To Long Integer(number=w276) -> (32bit integer=w275:i32)
                n107 = Bundle("Encoder position [selected units]"=w279, "Desired Position [selected units]"=w278) -> (→"Waveform Chart":T12)  [unwired: 1 in]
                n108 = call "Parse Xeryon STAT.vi"("STAT Word"=w275) -> ("STAT True"=→"STAT":string)  [unwired: 9 in, 1 out]
                n109 = Divide(x=w281, y=65536.0) -> (x/y=w283:dbl)
                n110 = Multiply(x=w283, y=16448250.0) -> (x*y=w280:dbl)
                n111 = To Unsigned Long Integer(number=w280) -> (unsigned 32bit integer=→"Color Box":u32)
              }
            }
            n112 = call <vilib>:"Add State(s) to Queue__jki_lib_state_machine.vi"("State(s) in (\"\")"=w272) -> ("States Out"=w271:string)  [unwired: 14 in]
          }
          frame "UI: Cursor Set" {
            # "Argument"
            # "Initialize the User Interface, here.\n(this is called automatically, by the Macro: Init)"
            n113 = disable-structure shown="Default" {
              disable-tunnel: w294 -> [w299 w302]
              disable-tunnel: [w299 w301] -> w293
              disable-tunnel: w292 -> [_ w300]
              frame condition #0 {
              }
              frame condition #1 (active) {
                n114 = case shown="\"Busy\"" w300 {
                  tunnel: w302 -> [w304 w306]
                  tunnel: [w303 w305] -> w301
                  frame "Idle", Default {
                    n115 = call <vilib>:"Unset Busy.vi"("error in (no error)"=w304) -> ("error out"=w303:errorcluster)  [unwired: 10 in]
                  }
                  frame "Busy" {
                    n116 = call <vilib>:"Set Busy.vi"("error in (no error)"=w306) -> ("error out"=w305:errorcluster)  [unwired: 9 in, 1 out]
                  }
                }
              }
            }
            n117 = call <vilib>:"Add State(s) to Queue__jki_lib_state_machine.vi"("State(s) in (\"\")"=w298) -> ("States Out"=w297:string)  [unwired: 14 in]
          }
          frame "UI: Front Panel State" {
            # "Argument"
            # "Set Front Panel Open or Closed\n(Usage: \"UI: Front Panel State >> Open|Close\")"
            n118 = Unbundle By Name(w310) -> ("Core.Current VI Reference"=w309:refnum<vi>)
            n119 = disable-structure shown="Default" {
              disable-tunnel: w312 -> [w318 w341]
              disable-tunnel: [w317 w341] -> w311
              disable-tunnel: w309 -> [w316 _]
              disable-tunnel: w308 -> [w315 _]
              frame condition #0 (active) {
                n120 = case shown="\"Close\"" w315 {
                  tunnel: w318 -> [w322 w335]
                  tunnel: [w324 w336] -> w317
                  tunnel: w316 -> [w323 w333]
                  frame "Open", Default {
                    n121 = property class="VI"(reference=w323, error in=w322) -> (reference out=w320:refnum<vi>, error out=w321:errorcluster, "FP.State"=w319:T6)
                    n122 = case shown="\"Closed\"" w319 {
                      tunnel: [w327 w330] -> w324
                      tunnel: w321 -> [w326 w330]
                      tunnel: w320 -> [w325 _]
                      frame "Closed" {
                        n123 = invoke class="VI" method="FP.Open"(reference=w325, error in=w326, "Activate"=TRUE, "State"=T6."Standard") -> (error out=w327:errorcluster)  [unwired: 1 in, 4 out]
                      }
                      frame Default {
                      }
                    }
                  }
                  frame "Close" {
                    n124 = property class="VI"(reference=w333, error in=w335) -> (reference out=w332:refnum<vi>, error out=w334:errorcluster, "FP.State"=w331:T6)
                    n125 = case shown="Default" w331 {
                      tunnel: [w337 w340] -> w336
                      tunnel: w334 -> [w337 w339]
                      tunnel: w332 -> [_ w338]
                      frame "Invalid", "Closed" {
                      }
                      frame Default {
                        n126 = invoke class="VI" method="FP.Close"(reference=w338, error in=w339) -> (error out=w340:errorcluster)  [unwired: 1 in, 2 out]
                      }
                    }
                  }
                }
              }
              frame condition #1 {
              }
            }
            n127 = call <vilib>:"Add State(s) to Queue__jki_lib_state_machine.vi"("State(s) in (\"\")"=w314) -> ("States Out"=w313:string)  [unwired: 14 in]
          }
          frame "---------- Macro ----------" {
            # "Do not put any code in this frame.\n(It is a separator no-op. You can make a copy of this frame to create a new Macro frame)"
            n128 = call <vilib>:"Add State(s) to Queue__jki_lib_state_machine.vi"("State(s) in (\"\")"=w346) -> ("States Out"=w345:string)  [unwired: 14 in]
          }
          frame "Macro: Initialize" {
            w349 = "UI: Initialize\nMacro: Read UI Config\nAction: Open\n//UI: Front Panel State >> Open"  # UI: Initialize Macro: Read UI Config Action: Open //UI: Front Panel State >> Open
            # "Initialization Macro\n(This is called once, when the VI starts)"
            n129 = call <vilib>:"Add State(s) to Queue__jki_lib_state_machine.vi"("State(s) in Front (\"\")"="Data: Initialize\nInitialize Core Data\nEvents: Register", "State(s) in (\"\")"="Process: Sync", "State(s) at Back (\"\")"=w349) -> ("States Out"=w348:string)  [unwired: 12 in]
            n130 = call <vilib>:"Add State(s) to Queue__jki_lib_state_machine.vi"("State(s) in Front (\"\")"=w348, "State(s) in (\"\")"=w355) -> ("States Out"=w354:string)  [unwired: 13 in]
          }
          frame "Macro: Post Error Handling" {
            # "Clear Last Error?"
            n131 = Unbundle By Name(w357) -> ("Core.Last Error.remaining states"=w359:string, "Core.Shutdown?"=w360:bool)
            n132 = Unbundle By Name(w357) -> ("Core.Last Error.error"=w363:errorcluster)
            n133 = case shown="False" FALSE {
              tunnel: w363 -> [w371 _]
              tunnel: [w371 _] -> w362
              frame False {
              }
              frame True {
              }
            }
            n134 = case shown="True" w360 {
              tunnel: w359 -> [w368 w370]
              tunnel: [w368 w369] -> w356
              frame False {
                # "These are the remaining states (at the moment the error occured). States can be altered according to business logic."
                # "NOT SHUTTING DOWN"
              }
              frame True {
                # "Developer can decide to alter the states but should be aware that during the shutdown process, there are certain states that must be run for the SMO to properly shut itself (and this process) down. As such, one can add states to perform additional clean-ups, but should append the remaining state to be executed."
                # "SHUTTING DOWN"
                n135 = call <vilib>:"Add State(s) to Queue__jki_lib_state_machine.vi"("State(s) in (\"\")"=w370) -> ("States Out"=w369:string)  [unwired: 14 in]
              }
            }
            n136 = Bundle By Name(cluster=w357, "Core.Last Error.error"=w362) -> (w358:T10)
            n137 = call <vilib>:"Add State(s) to Queue__jki_lib_state_machine.vi"("State(s) in Front (\"\")"=w356, "State(s) in (\"\")"=w367) -> ("States Out"=w366:string)  [unwired: 13 in]
          }
          frame "Macro: Read UI Config" {
            # "Do not put any code in this frame.\n(It is a separator no-op. You can make a copy of this frame to create a new Macro frame)"
            n138 = call <vilib>:"Add State(s) to Queue__jki_lib_state_machine.vi"("State(s) in Front (\"\")"="Configuration: Initialize\nConfiguration: Read UI Config File\nUI: Update FP Controls" ("State(s) in Front (\"\")"), "State(s) in (\"\")"=w377) -> ("States Out"=w376:string)  [unwired: 13 in]
          }
          frame "Macro: Write UI Config" {
            # "Do not put any code in this frame.\n(It is a separator no-op. You can make a copy of this frame to create a new Macro frame)"
            n139 = call <vilib>:"Add State(s) to Queue__jki_lib_state_machine.vi"("State(s) in Front (\"\")"="Data: Set UI Cluster\nConfiguration: Write UI Config File" ("State(s) in Front (\"\")"), "State(s) in (\"\")"=w383) -> ("States Out"=w382:string)  [unwired: 13 in]
          }
          frame "Macro: Exit" {
            # "Exit Macro\n(This is called once, when the VI exits)"
            n140 = Unbundle By Name(w385) -> ("Core.Close Panel on Exit?"=w395:bool)
            n141 = Select(t="UI: Front Panel State >> Close", s=w395, f="" ("Empty String Constant")) -> (s? t:f=w392:string)
            n142 = call <vilib>:"Add State(s) to Queue__jki_lib_state_machine.vi"("State(s) in Front (\"\")"="Data: Cleanup\nEvents: Unregister\nProcess: Self Terminate", "State(s) in (\"\")"="Process: Sync", "State(s) at Back (\"\")"="Exit") -> ("States Out"=w387:string)  [unwired: 12 in]
            n143 = call <vilib>:"Add State(s) to Queue__jki_lib_state_machine.vi"("State(s) in Front (\"\")"="Action: Close\nMacro: Write UI Config", "State(s) in (\"\")"=w392, "State(s) at Back (\"\")"=w387) -> ("States Out"=w391:string)  [unwired: 12 in]
            n144 = call <vilib>:"Add State(s) to Queue__jki_lib_state_machine.vi"("State(s) in Front (\"\")"=w391, "State(s) in (\"\")"=w398) -> ("States Out"=w397:string)  [unwired: 13 in]
          }
          frame "---------- Process ----------" {
            # "Template Separator\n(You can make a copy of, or modify, this frame)"
            n145 = call <vilib>:"Add State(s) to Queue__jki_lib_state_machine.vi"("State(s) in (\"\")"=w403) -> ("States Out"=w402:string)  [unwired: 14 in]
          }
          frame "Process: Sync" {
            n146 = Unbundle By Name(w411) -> ("Instrument UI"=w407:refnum<class "Inst UI.Xeryon-Rotator.lvclass">)
            n147 = call <vilib>:"WaitOnProcessSync.vi"("error in (no error)"=w406, "SMO"=w407) -> ("error out"=w405:errorcluster, "Don't run?"=w410:bool)  [unwired: 7 in, 1 out]
            n148 = Select(t="Data: Cleanup\nEvents: Unregister\nExit", s=w410, f="" ("Empty String Constant")) -> (s? t:f=w404:string)
            n149 = call <vilib>:"Add State(s) to Queue__jki_lib_state_machine.vi"("State(s) in Front (\"\")"=w404, "State(s) in (\"\")"=w414) -> ("States Out"=w413:string)  [unwired: 13 in]
          }
          frame "Process: Self Terminate" {
            n150 = Unbundle By Name(w416) -> ("Instrument UI"=w415:refnum<class "Inst UI.Xeryon-Rotator.lvclass">)
            n151 = call <vilib>:"SelfTerminate.vi"("error in (no error)"=w418, "SMO in"=w415) -> ("error out"=w417:errorcluster)  [unwired: 8 in, 1 out]
            n152 = call <vilib>:"Add State(s) to Queue__jki_lib_state_machine.vi"("State(s) in (\"\")"=w421) -> ("States Out"=w420:string)  [unwired: 14 in]
          }
          frame "---------- Events ----------" {
            # "Template Separator\n(You can make a copy of, or modify, this frame)"
            n153 = call <vilib>:"Add State(s) to Queue__jki_lib_state_machine.vi"("State(s) in (\"\")"=w426) -> ("States Out"=w425:string)  [unwired: 14 in]
          }
          frame "Events: Register" {
            # "Expand to add\nmore events"
            # "Base Class Protected Events"
            n154 = Unbundle By Name(w440) -> ("Instrument UI"=w433:refnum<class "Inst UI.Xeryon-Rotator.lvclass">, "Instrument"=w432:refnum<class "Inst.Xeryon-Rotator.lvclass">)
            n155 = call <vilib>:"GetProtectedEvents.vi"("SMO"=w433) -> ("error out"=w436:errorcluster, "SMO Protected Events"=w438:T13)  [unwired: 8 in, 1 out]
            n156 = call <userlib>:"Instrument.GetPublicEvents.vi"("Instrument"=w432) -> ("error out"=w434:errorcluster, "Instrument Public Events"=w435:T14, "Instrument out"=w430:refnum<class "Inst.Xeryon-Rotator.lvclass">)  [unwired: 8 in]
            n157 = call "Inst.Xeryon-Rotator.GetPublicEvents.vi"("Inst.Xeryon-Rotator in"=w430) -> ("error out"=w429:errorcluster, "Inst.Xeryon-Rotator Public Events"=w431:T15)  [unwired: 8 in, 1 out]
            n158 = register-events(w438, w435, w431) -> (reference out=w439:refnum<event-registration>, error out=w428:errorcluster)  [unwired: 2 in]
            n159 = Merge Errors(w428, w429, w434, w436, w427) -> (w437:errorcluster)
            n160 = call <vilib>:"Add State(s) to Queue__jki_lib_state_machine.vi"("State(s) in (\"\")"=w442) -> ("States Out"=w441:string)  [unwired: 14 in]
          }
          frame "Events: Unregister" {
            n161 = Unregister For Events(event registration refnum=w445, error in=w444) -> (error out=w443:errorcluster)
            n162 = call <vilib>:"Add State(s) to Queue__jki_lib_state_machine.vi"("State(s) in (\"\")"=w448) -> ("States Out"=w447:string)  [unwired: 14 in]
          }
          frame "---------- Configuration ----------" {
            # "Do not put any code in this frame.\n(It is a separator no-op. You can make a copy of this frame to create a new UI frame)"
            n163 = call <vilib>:"Add State(s) to Queue__jki_lib_state_machine.vi"("State(s) in (\"\")"=w453) -> ("States Out"=w452:string)  [unwired: 14 in]
          }
          frame "Configuration: Initialize" {
            # "Do not put any code in this frame.\n(It is a separator no-op. You can make a copy of this frame to create a new UI frame)"
            n164 = Unbundle By Name(w461) -> ("Configuration"=w459:refnum<class "Configuration.lvclass">, "Instrument"=w460:refnum<class "Inst.Xeryon-Rotator.lvclass">)
            n165 = call <vilib>:"GetName.vi"("error in (no error)"=w463, "SMO"=w460) -> ("error out"=w462:errorcluster, "Name"=w464:string)  [unwired: 6 in, 2 out]
            n166 = call <userlib>:"Default Path.vi"("error in (no error)"=w462, "Folder Name [Application Name]"=w464, "Configuration in"=w459) -> ("error out"=w455:errorcluster, "Configuration out"=w458:refnum<class "Configuration.lvclass">)  [unwired: 7 in]
            n167 = call <userlib>:"Write Section.vi"("error in (no error)"=w455, "Section"="UI", "Configuration in"=w458) -> ("error out"=w454:errorcluster, "Configuration out"=w457:refnum<class "Configuration.lvclass">)  [unwired: 7 in]
            n168 = Bundle By Name(cluster=w461, "Configuration"=w457) -> (w465:T10)
            n169 = call <vilib>:"Add State(s) to Queue__jki_lib_state_machine.vi"("State(s) in (\"\")"=w468) -> ("States Out"=w467:string)  [unwired: 14 in]
          }
          frame "Configuration: Write UI Config File" {
            # "Do not put any code in this frame.\n(It is a separator no-op. You can make a copy of this frame to create a new Data frame)"
            n170 = Unbundle By Name(w473) -> ("Configuration"=w470:refnum<class "Configuration.lvclass">, "UI Cluster"=w472:T8)
            n171 = call <userlib>:"Write Configuration.vi"("error in (no error)"=w469, "Variant"=w472, "Configuration in"=w470) -> ("error out"=w471:errorcluster)  [unwired: 7 in, 1 out]
            n172 = call <vilib>:"Add State(s) to Queue__jki_lib_state_machine.vi"("State(s) in (\"\")"=w476) -> ("States Out"=w475:string)  [unwired: 14 in]
          }
          frame "Configuration: Read UI Config File" {
            # "Do not put any code in this frame.\n(It is a separator no-op. You can make a copy of this frame to create a new UI frame)"
            n173 = Unbundle By Name(w479) -> ("UI Cluster"=w482:T8, "Configuration"=w485:refnum<class "Configuration.lvclass">)
            n174 = call <userlib>:"Read Configuration.vi"("INI Fomatted Cluster Type"=w482, "error in (no error)"=w481, "Configuration in"=w485) -> ("error out"=w484:errorcluster, "Configuration"=w483:variant)  [unwired: 6 in, 1 out]
            n175 = Variant To Data(error in=w484, type=w482, Variant=w483) -> (data=w478:T8, error out=w480:errorcluster)
            n176 = Bundle By Name(cluster=w479, "UI Cluster"=w478) -> (w477:T10)
            n177 = call <vilib>:"Add State(s) to Queue__jki_lib_state_machine.vi"("State(s) in (\"\")"=w488) -> ("States Out"=w487:string)  [unwired: 14 in]
          }
          frame "---------- Action ----------" {
            n178 = Unbundle By Name(w490) -> ("Instrument"=w491:refnum<class "Inst.Xeryon-Rotator.lvclass">)
            n179 = Bundle By Name(cluster=w490, "Instrument"=w491) -> (w489:T10)
            n180 = call <vilib>:"Add State(s) to Queue__jki_lib_state_machine.vi"("State(s) in (\"\")"=w495) -> ("States Out"=w494:string)  [unwired: 14 in]
          }
          frame "Action: Notify UI Closed" {
            # "Notify that the UI has been closed"
            n181 = Unbundle By Name(w496) -> ("Instrument UI"=w499:refnum<class "Inst UI.Xeryon-Rotator.lvclass">)
            n182 = call <vilib>:"Hide.vi"("error in (no error)"=w498, "SMO.UI"=w499) -> ("error out"=w497:errorcluster)  [unwired: 8 in, 1 out]
            n183 = call <vilib>:"Add State(s) to Queue__jki_lib_state_machine.vi"("State(s) in (\"\")"=w502) -> ("States Out"=w501:string)  [unwired: 14 in]
          }
          frame "Action: getAll" {
            n184 = Unbundle By Name(w509) -> ("getAll"=w507:T5, "Instrument"=w512:refnum<class "Inst.Xeryon-Rotator.lvclass">)
            n185 = call <userlib>:"getAll.vi"("error in (no error)"=w510, "Instrument in"=w512) -> ("error out"=w504:errorcluster, "getAll"=w506:variant, "Instrument out"=w508:refnum<class "Inst.Xeryon-Rotator.lvclass">)  [unwired: 7 in]
            n186 = call "JSON to LVtype.vim"("type"=w507, "error in (no error)"=w504, "JSON Data in"=w506) -> ("error out"=w503:errorcluster, "Data out"=w505:T5)  [unwired: 7 in]
            n187 = Bundle By Name(cluster=w509, "Instrument"=w508, "getAll"=w505) -> (w511:T10)
            n188 = call <vilib>:"Add State(s) to Queue__jki_lib_state_machine.vi"("State(s) in Front (\"\")"="" ("State(s) in Front (\"\")"), "State(s) in (\"\")"=w516) -> ("States Out"=w515:string)  [unwired: 13 in]
          }
          frame "Action: Open" {
            n189 = Unbundle By Name(w523) -> ("Instrument"=w521:refnum<class "Inst.Xeryon-Rotator.lvclass">)
            n190 = call <userlib>:"Write Client Type.vi"("error in (no error)"=w518, "Client Type [Remote]"=Client_Type--Enum."Local" ("Client Type"), "Instrument in"=w521) -> ("error out"=w519:errorcluster, "Instrument out"=w520:refnum<class "Inst.Xeryon-Rotator.lvclass">)  [unwired: 7 in]
            n191 = call-dynamic "Open.vi"("error in (no error)"=w519, "Inst.Xeryon-Rotator in"=w520) -> ("error out"=w526:errorcluster, "Inst.Xeryon-Rotator out"=w522:refnum<class "Inst.Xeryon-Rotator.lvclass">)  [unwired: 8 in]
            n192 = Bundle By Name(cluster=w523, "Instrument"=w522) -> (w524:T10)
            n193 = call <vilib>:"Add State(s) to Queue__jki_lib_state_machine.vi"("State(s) in Front (\"\")"="" ("State(s) in Front (\"\")"), "State(s) in (\"\")"=w529) -> ("States Out"=w528:string)  [unwired: 13 in]
          }
          frame "Action: Close" {
            n194 = Unbundle By Name(w531) -> ("Instrument"=w534:refnum<class "Inst.Xeryon-Rotator.lvclass">)
            n195 = call-dynamic "Close.vi"("error in (no error)"=w532, "Inst.Xeryon-Rotator in"=w534) -> ("error out"=w536:errorcluster, "Inst.Xeryon-Rotator out"=w530:refnum<class "Inst.Xeryon-Rotator.lvclass">)  [unwired: 8 in]
            n196 = Bundle By Name(cluster=w531, "Instrument"=w530) -> (w533:T10)
            n197 = call <vilib>:"Add State(s) to Queue__jki_lib_state_machine.vi"("State(s) in Front (\"\")"="" ("State(s) in Front (\"\")"), "State(s) in (\"\")"=w539) -> ("States Out"=w538:string)  [unwired: 13 in]
          }
          frame "Action: Send Message to Instrument" {
            # "Send a message (command, data, etc) to the Instrument:process.vi"
            n198 = Unbundle By Name(w546) -> ("Instrument"=w545:refnum<class "Inst.Xeryon-Rotator.lvclass">, "Message.Command"=w541:string, "Message.Data"=w540:variant)
            n199 = call-poly <userlib>:"Instrument.sendMessageToProcess.vi"("error in (no error)"=w543, "Data"=w540, "Command"=w541, "Instrument"=w545) -> ("error out"=w542:errorcluster, "Instrument"=w544:refnum<class "Inst.Xeryon-Rotator.lvclass">)  [unwired: 6 in]
            n200 = Bundle By Name(cluster=w546, "Instrument"=w544) -> (w547:T10)
            n201 = call <vilib>:"Add State(s) to Queue__jki_lib_state_machine.vi"("State(s) in Front (\"\")"="" ("State(s) in Front (\"\")"), "State(s) in (\"\")"=w551) -> ("States Out"=w550:string)  [unwired: 13 in]
          }
          frame "Action: Send Message to Child" {
            # "Send a message (command, data, etc) to the Instrument.Child:process.vi"
            n202 = Unbundle By Name(w558) -> ("Instrument"=w557:refnum<class "Inst.Xeryon-Rotator.lvclass">, "Message.Command"=w553:string, "Message.Data"=w552:variant)
            n203 = call "Inst.Xeryon-Rotator.MessageToProcess.vi"("error in (no error)"=w555, "Data"=w552, "Command"=w553, "Inst.Xeryon-Rotator in"=w557) -> ("error out"=w554:errorcluster, "Inst.Xeryon-Rotator out"=w556:refnum<class "Inst.Xeryon-Rotator.lvclass">)  [unwired: 6 in]
            n204 = Bundle By Name(cluster=w558, "Instrument"=w556) -> (w559:T10)
            n205 = call <vilib>:"Add State(s) to Queue__jki_lib_state_machine.vi"("State(s) in Front (\"\")"="" ("State(s) in Front (\"\")"), "State(s) in (\"\")"=w563) -> ("States Out"=w562:string)  [unwired: 13 in]
          }
        }
      }
    }
    frame Error {
    }
  }
  n206 = call-parent "Process.vi"("error in"=w5, "Instrument UI in"=w4) -> ("error out"=w2:errorcluster, "Instrument UI out"=→"Inst UI.Xeryon-Rotator out":refnum<class "Inst UI.Xeryon-Rotator.lvclass">)  [unwired: 8 in]
  n207 = Merge Errors(w2, w1) -> (→"error out":errorcluster)
